vi "Instrument.PPMS2.Write Configuration File.vi"(8 "error in (no error)":errorcluster, 11 "instrument.PPMS2 in":refnum<class "instrument.PPMS2.lvclass">) -> (0 "error out":errorcluster, 3 "instrument.PPMS2 out":refnum<class "instrument.PPMS2.lvclass">)   [LabVIEW 2016, in "instrument.PPMS2.lvclass"]
uses:
  instrument.PPMS2.lvclass
  C:/Program Files (x86)/National Instruments/LabVIEW 2016/user.lib/LevyLab/Levylab Instruments/SMOs/Instrument/Instrument.lvclass
  <userlib>/LevyLab/Levylab Instruments/SMOs/Instrument/Instrument.lvclass/Instrument.ctl
  instrument.PPMS2.lvclass/instrument.PPMS2.ctl
  <userlib>/LevyLab/Levylab Instruments/SMOs/Configuration/Configuration.lvclass
  <userlib>/LevyLab/Levylab Instruments/SMOs/Instrument/Instrument.lvclass
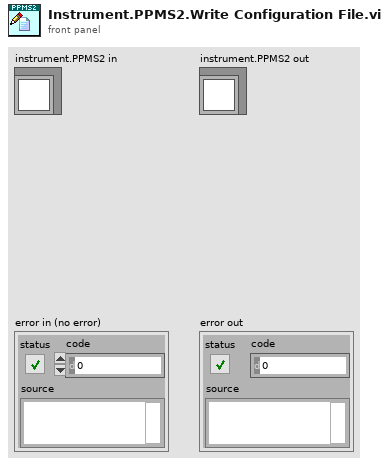
[diagram p1: front panel]
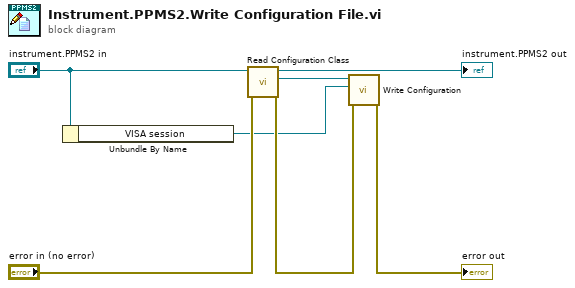
[diagram p0: block diagram]
diagram:
  n1 = Unbundle By Name("instrument.PPMS2 in") -> ("VISA session"=w1:refnum<visa-resource-name>)
  n2 = call <userlib>:"Read Configuration Class.vi"("error in (no error)"="error in (no error)", "Instrument in"="instrument.PPMS2 in") -> ("error out"=w5:errorcluster, "Configuration.lvclass"=w6:refnum<class "Configuration.lvclass">, "Instrument out"=→"instrument.PPMS2 out":refnum<class "instrument.PPMS2.lvclass">)  [unwired: 7 in]
  n3 = call <userlib>:"Write Configuration.vi"("error in (no error)"=w5, "Variant"=w1, "Configuration in"=w6) -> ("error out"=→"error out":errorcluster)  [unwired: 7 in, 1 out]
